vi "CT_SaveMultiWaveformBinary.vi"(1 "error in (no error)":errorcluster, 3 "waveforms":waveform(dbl)[][](array[waveform]), 4 "file path (dialog if empty)":path) -> (0 "error out":errorcluster)   [LabVIEW 2009]
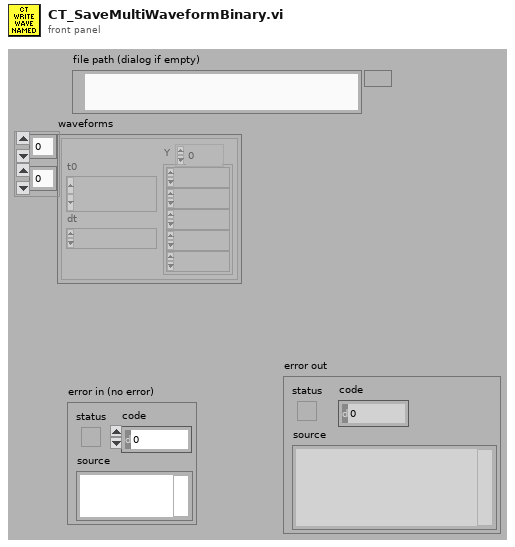
[diagram p1: front panel]
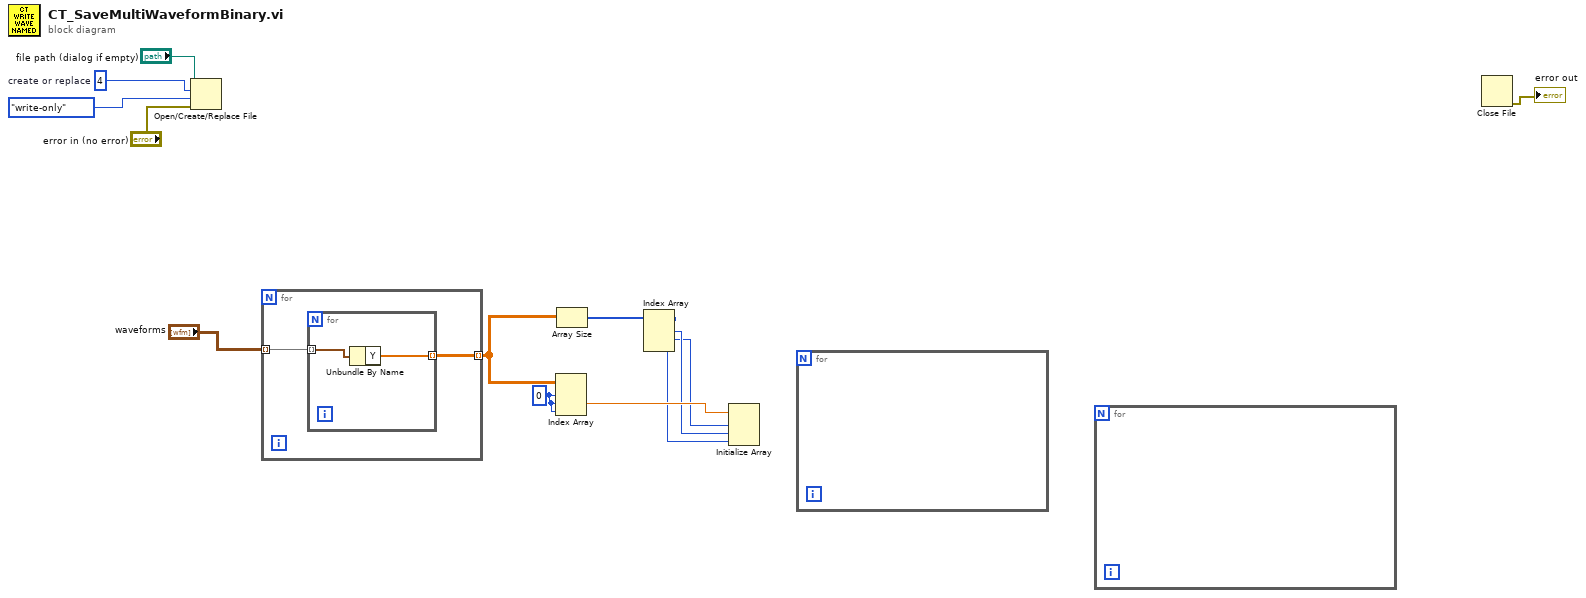
[diagram p0: block diagram]
diagram:
  w6 = 0 ("index (page)")
  w12 = i16 4  # create or replace
  n1 = Open/Create/Replace File(file path (use dialog)="file path (dialog if empty)", error in="error in (no error)", operation (0:open)=w12, access (0:read/write)=enum16{"read/write", "read-only", "write-only"}."write-only") -> (refnum out=w10:refnum<file>, error out=w9:errorcluster)  [unwired: 2 in, 1 out]
  n2 = for {
    tunnel: "waveforms" -> [w19] mode=indexing
    tunnel: [w18] -> w7 mode=indexing
    n3 = for {
      tunnel: w19 -> [w21] mode=indexing
      tunnel: [w20] -> w18 mode=indexing
      n4 = Unbundle By Name(w21) -> ("Y"=w20:dbl[])
    }
  }
  n5 = Index Array(array=w7, index (dim 0)=w6, index (dim 1)=w6, index (dim 2)=w6) -> (element=w4:dbl)
  n6 = Array Size(array=w7) -> (size(s)=w5:i32[])
  n7 = Index Array(array=w5) -> (element #1=w3:i32, element #2=w2:i32, element #3=w1:i32)  [unwired: 3 in]
  n8 = Initialize Array(w4, w2, w3, w1) -> ()  [unwired: 1 out]
  n9 = for {
  }
  n10 = for {
  }
  n11 = Close File() -> (error out=→"error out":errorcluster, refnum=w16:refnum<file>, error in=w15:errorcluster)  [unwired: 1 out]
